vi "Module API.vi"(8 "error in (no error)":errorcluster, 11 "Module in":refnum<class "Module.lvclass">) -> (0 "error out":errorcluster, 2 "API":refnum<class "API.lvclass">, 3 "Module out":refnum<class "Module.lvclass">)   [LabVIEW 2020]
uses:
  Module.lvclass
  API/API.lvclass
  Module.lvclass/Module.ctl
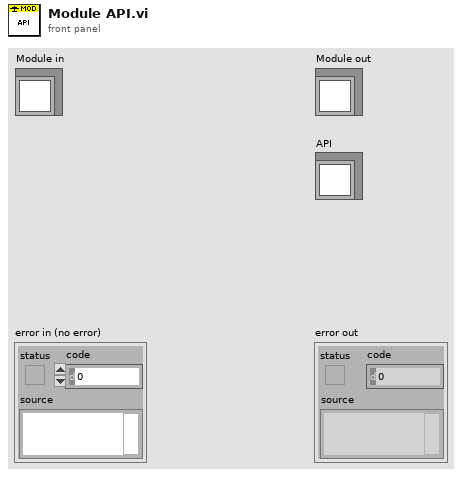
[diagram p1: front panel]
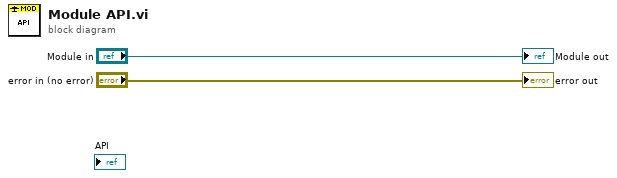
[diagram p0: block diagram]
diagram:
  "error out" <- "error in (no error)"
  "Module out" <- "Module in"
